vi "Check if LineScan settings and LineScan image.vi"() -> (2 "LineScan Image?":bool, 3 "LineScan settings?":bool)   [LabVIEW 2012]
uses:
  Custom Controls/Image Types.ctl
  Custom Controls/scan mode main settings tab.ctl
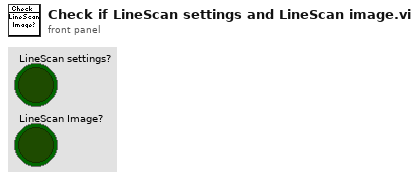
[diagram p1: front panel]
types:
  T1 = typedef "scan mode main settings tab.ctl" = enum32{"2D frame", "2D line scan", "general settings", "Z Stack", "piezo"}
  T2 = typedef "Image Types.ctl" = enum16{"Frame Scan", "Line Scan", "RGB Overlay", "ROI", "All Channels Frame"}
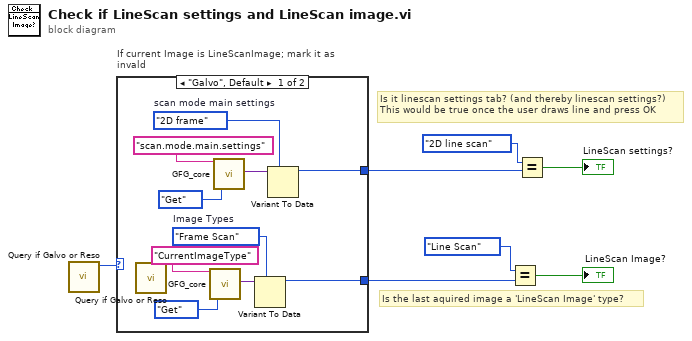
[diagram p0: block diagram]
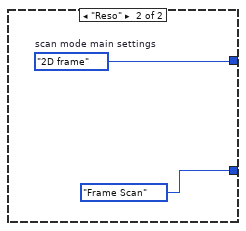
[diagram p2: hidden frame]
diagram:
  # "Is the last aquired image a 'LineScan Image' type?"
  # "Is it linescan settings tab? (and thereby linescan settings?)\nThis would be true once the user draws line and press OK"
  n1 = call "Query if Galvo or Reso.vi"() -> ("System Type"=w7:enum16{"Galvo", "Reso"})  [unwired: 10 in, 1 out]
  n2 = case "If current Image is LineScanImage; mark it as invald" shown="\"Galvo\", Default" w7 {
    tunnel: [w14 Image_Types."Frame Scan" ("Image Types")] -> w5
    tunnel: [w9 w18] -> w4
    frame "Galvo", Default {
      w8 = scan_mode_main_settings_tab."2D frame"  # scan mode main settings
      w13 = Image_Types."Frame Scan"  # Image Types
      n3 = call "GFG_core.vi"("Variable Name in"="CurrentImageType", "Action"=enum16{"Init", "Set", "Get", "Clear"}."Get") -> ("Variant Out"=w15:variant)  [unwired: 11 in, 6 out]
      n4 = call "GFG_core.vi"("Variable Name in"="scan.mode.main.settings", "Action"=enum16{"Init", "Set", "Get", "Clear"}."Get") -> ("Variant Out"=w10:variant)  [unwired: 11 in, 6 out]
      n5 = Variant To Data(type=w13, Variant=w15) -> (data=w14:T2)  [unwired: 1 in, 1 out]
      n6 = Variant To Data(type=w8, Variant=w10) -> (data=w9:T1)  [unwired: 1 in, 1 out]
    }
    frame "Reso" {
      w18 = scan_mode_main_settings_tab."2D frame"  # scan mode main settings
    }
  }
  n7 = call "Query if Galvo or Reso.vi"() -> ()  [unwired: 10 in, 2 out]
  n8 = Equal?(x=Image_Types."Line Scan", y=w5) -> (x = y?=→"LineScan Image?":bool)
  n9 = Equal?(x=scan_mode_main_settings_tab."2D line scan", y=w4) -> (x = y?=→"LineScan settings?":bool)
